vi "Swerve Drive.vi"(0 "Drive Joystick":string="My Joystick RefNum") -> ()   [LabVIEW 2018]
uses:
  <vilib>/Rock Robotics/Network Tables/NT Write Number.vi
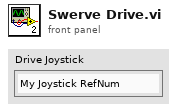
[diagram p1: front panel]
types:
  T1 = cluster{"RR Offset":dbl, "FR Offset":dbl, "RL Offset":dbl, "FL Offset":dbl}
  T2 = typedef "Encoder Data.ctl" = cluster{"RR Angle":dbl, "FR Angle":dbl, "RL Angle":dbl, "FL Angle":dbl}
  T3 = typedef "Kinematics Data.ctl" = cluster{"RR Drive Power":dbl, "FR Drive Power":dbl, "RL Drive Power":dbl, "FL Drive Power":dbl, "RR Steer Angle":dbl, "FR Steer Angle":dbl, "RL Steer Angle":dbl, "FL Steer Angle":dbl}
  T4 = typedef "Error Data.ctl" = cluster{"RR Error":dbl, "FR Error":dbl, "RL Error":dbl, "FL Error":dbl}
  T5 = typedef "Motor Data.ctl" = cluster{"RR Drive Power":dbl, "FR Drive Power":dbl, "RL Drive Power":dbl, "FL Drive Power":dbl}
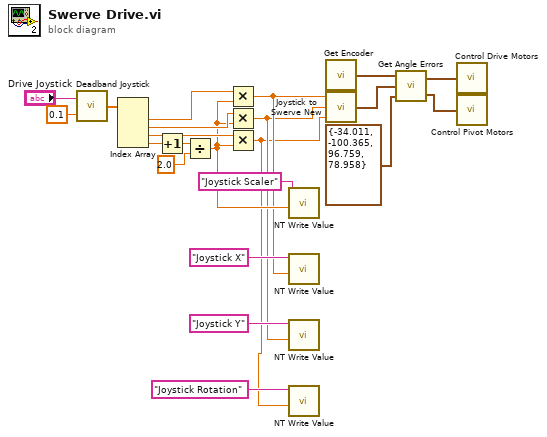
[diagram p0: block diagram]
diagram:
  n1 = call "Deadband Joystick.vi"("Deadband Amount"=0.1, "Joystick"="Drive Joystick") -> ("Deadbanded Axes"=w20:dbl[])
  n2 = Index Array(array=w20) -> (element #1=w16:dbl, element #2=w15:dbl, element #3=w14:dbl, element #4=w19:dbl)  [unwired: 4 in]
  n3 = Increment(x=w19) -> (x+1=w18:dbl)
  n4 = Divide(x=w18, y=2.0) -> (x/y=w13:dbl)
  n5 = Multiply(x=w16, y=w13) -> (x*y=w8:dbl)
  n6 = Multiply(x=w15, y=w13) -> (x*y=w7:dbl)
  n7 = Multiply(x=w14, y=w13) -> (x*y=w6:dbl)
  n8 = call-poly <vilib>:"NT Write Value.vi"("Numeric"=w13, "Name"="Joystick Scaler") -> ()  [unwired: 9 in, 1 out]
  n9 = call-poly <vilib>:"NT Write Value.vi"("Numeric"=w8, "Name"="Joystick X") -> ()  [unwired: 9 in, 1 out]
  n10 = call-poly <vilib>:"NT Write Value.vi"("Numeric"=w7, "Name"="Joystick Y") -> ()  [unwired: 9 in, 1 out]
  n11 = call-poly <vilib>:"NT Write Value.vi"("Numeric"=w6, "Name"="Joystick Rotation") -> ()  [unwired: 9 in, 1 out]
  n12 = call "Get Encoder.vi"() -> ("Encoder Data"=w4:T2)
  n13 = call "Joystick to Swerve New.vi"("Joystick Y"=w6, "Joystick R"=w7, "Joystick X"=w8) -> ("Kinematics Data"=w3:T3)
  n14 = call "Get Angle Errors.vi"("Offsets"=T1 {"RR Offset"=-34.011, "FR Offset"=-100.365, "RL Offset"=96.759, "FL Offset"=78.958}, "Kinematics Data"=w3, "Encoder Data"=w4) -> ("Angle Errors"=w1:T4, "Drive Powers"=w2:T5)
  n15 = call "Control Drive Motors.vi"("Motor Speeds"=w2) -> ()
  n16 = call "Control Pivot Motors.vi"("Angle Errors"=w1) -> ()
